vi "IEI.vi"() -> ()   [LabVIEW 2015]
panel:
  out "Output (flattened)":string="1\t10\t100\n2\t11\t110\n3\t12\t120\n4\t13\t130\n5\t14\t140\n6\t15\t150\n7\t16\t160\n8\t17\t170\n9\t18\t180\n"
  in  "Input (flattened)":string="1\t10\t100\n2\t11\t110\n3\t12\t120\n4\t13\t130\n5\t14\t140\n6\t15\t150\n7\t16\t160\n8\t17\t170\n9\t18\t180\n"
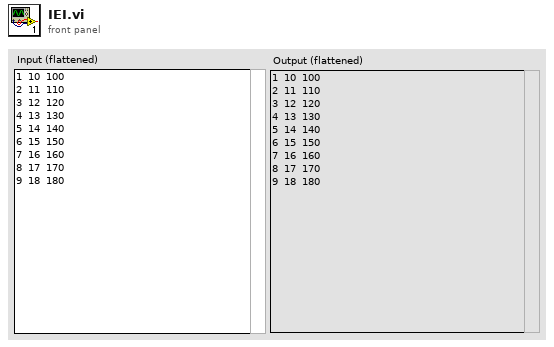
[diagram p1: front panel]
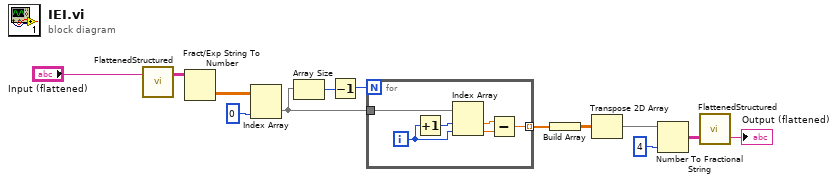
[diagram p0: block diagram]
diagram:
  n1 = call <userlib>:"FlattenedStructured.vi"("Input (flattened)"="Input (flattened)") -> ("Output (stuctured)"=w12:string[][])  [unwired: 1 in, 1 out]
  n2 = Fract/Exp String To Number(string=w12) -> (number=w11:dbl[][])  [unwired: 3 in, 1 out]
  n3 = Index Array(array=w11, index (col)=0 ("비활성화된 인덱스 (열)")) -> (element=w7:dbl[])  [unwired: 1 in]
  n4 = Array Size(array=w7) -> (size(s)=w8:i32)
  n5 = Decrement(x=w8) -> (x-1=w9:i32)
  n6 = for {
    N: w9 -> [_]
    tunnel: w7 -> [w19]
    tunnel: [w14] -> w6 mode=indexing
    i -> [w17]
    n7 = Increment(x=w17) -> (x+1=w18:i32)
    n8 = Index Array(array=w19, index #1=w18, index #2=w17) -> (element #1=w16:dbl, element #2=w15:dbl)
    n9 = Subtract(x=w16, y=w15) -> (x-y=w14:dbl)
  }
  n10 = Build Array(w6) -> (w5:dbl[][])
  n11 = Transpose 2D Array(2D array=w5) -> (transposed array=w4:dbl[][])
  n12 = Number To Fractional String(number=w4, precision (6)=i16 4 ("정밀도(6)")) -> (F-format string=w3:string[][])  [unwired: 2 in]
  n13 = call <userlib>:"FlattenedStructured.vi"("Input (structured)"=w3) -> ("Output (flattened)"=→"Output (flattened)":string)  [unwired: 1 in, 1 out]
